vi "Set PORT step.vi"(8 "error in (no error)":errorcluster, 9 "v (0.000000)":dbl, 10 "i (0)":T1, 11 "VISA resource name":refnum<visa-resource-name>) -> (0 "error out":errorcluster, 3 "VISA resource name out":refnum<visa-resource-name>)   [LabVIEW 2009, in "SR400.lvlib"]
doc: "PY i { ,v }\nThe PY command sets and reads the PORT1 and\nPORT2 scan steps. i=1 or 2 to select PORT1 or\nPORT 2 and is required. If v is included, the scan\nstep is set to v Volts where -0.500 <= v <= 0.500.\nThe resolution is 0.005 V (5 mV). If v is absent,\nthe scan step is returned. The scan step may be set\nand read even if the selected port is in the FIXED\nmode. Changing the scan step during a scan will affect the level for the next count period and all\nthose that follow."
uses:
  SR400.lvlib
  Typedefs.llb/PORT Output.ctl
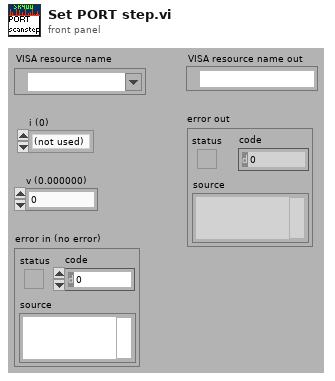
[diagram p1: front panel]
types:
  T1 = typedef "SR400.lvlib/PORT Output.ctl" = enum16{"(not used)", "PORT 1", "PORT 2"}
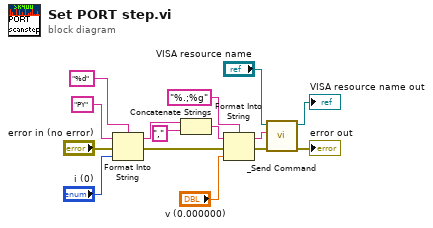
[diagram p0: block diagram]
diagram:
  n1 = Format Into String(format string="%d", initial string="PY" ("command"), error in="error in (no error)", "i (0)") -> (resulting string=w12:string, error out=w13:errorcluster)
  n2 = Concatenate Strings(w12, "," ("command")) -> (w7:string)
  n3 = Format Into String(format string="%.;%g", initial string=w7, error in=w13, "v (0.000000)") -> (resulting string=w4:string, error out=w3:errorcluster)
  n4 = call "_Send Command.vi"("error in (no error)"=w3, "Command"=w4, "VISA resource name"="VISA resource name") -> ("error out"=→"error out":errorcluster, "VISA resource name out"=→"VISA resource name out":refnum<visa-resource-name>)  [unwired: 1 in, 6 out]
